vi "Instrument Write to Log.vi"(8 "error in (no error)":errorcluster, 9 "Comment":string, 10 "Current VI's Path":path, 11 "Insstrument Address":refnum<visa-resource-name>) -> (0 "error out":errorcluster)   [LabVIEW 2018]
uses:
  Generic Reuse/Logger/Log File Input.ctl
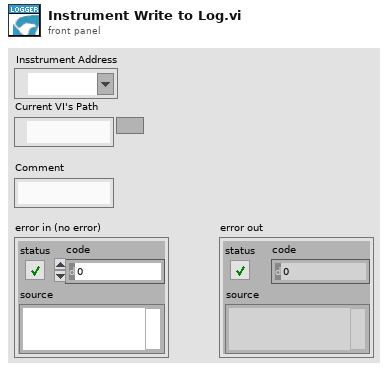
[diagram p1: front panel]
types:
  T1 = typedef "Log File Input.ctl" = cluster{"Log File Input":string, "Log Entry Type":enum16{"STANDARD", "WARNING", "CRITICAL"}}
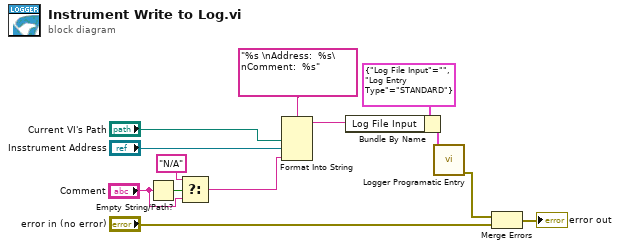
[diagram p0: block diagram]
diagram:
  n1 = Empty String/Path?(string/path="Comment") -> (empty?=w4:bool)
  n2 = Select(t="N/A", s=w4, f="Comment") -> (s? t:f=w2:string)
  n3 = Format Into String(format string="%s \nAddress:  %s\nComment:  %s", "Current VI's Path", "Insstrument Address", w2) -> (resulting string=w11:string)  [unwired: 2 in, 1 out]
  n4 = Bundle By Name(cluster=T1 {"Log File Input"="", "Log Entry Type"=enum."STANDARD"} ("Log File Input"), "Log File Input"=w11) -> (w13:T1)
  n5 = call "Logger Programatic Entry.vi"("Log File Input"=w13) -> ("error out"=w9:errorcluster)  [unwired: 14 in]
  n6 = Merge Errors(w9, "error in (no error)") -> (→"error out":errorcluster)
